vi "Request Frame.vi"(7 "Ignore Response":bool, 8 "error in (no error)":errorcluster, 9 "DA":u8, 10 "PGN":u32, 11 "Connection Info":T1) -> (0 "error out":errorcluster, 2 "Response Frame":T3 {"payload" format="%x"; "timestamp" format="%<%.7X\n%x>T"; "type" items=["CAN Data"=0, "CAN Remote"=1, "CAN Bus Error"=2, "CAN 2.0 Data"=8, "CAN FD Data"=16, "CAN FD+BRS Data"=24, "J1939 Data"=192, "Delay"=224, "Log Trigger"=225, "Start Trigger"=226]; "identifier" format="%x"}, 3 "Connection Info Out":T1)   [LabVIEW 2015, in "J1939 Addon Shared.lvlib"]
uses:
  J1939 Addon Shared.lvlib
  <vilib>/xnet/xnet.llb/XNET Frame CAN.ctl
  <vilib>/xnet/xnet.llb/XNET Frame Type CAN.ctl
  STM/TCP/stm_TCP Connection Info.ctl
  STM/_SubVIs/stm_MetaDataElement.ctl
  Types/Request Message.ctl
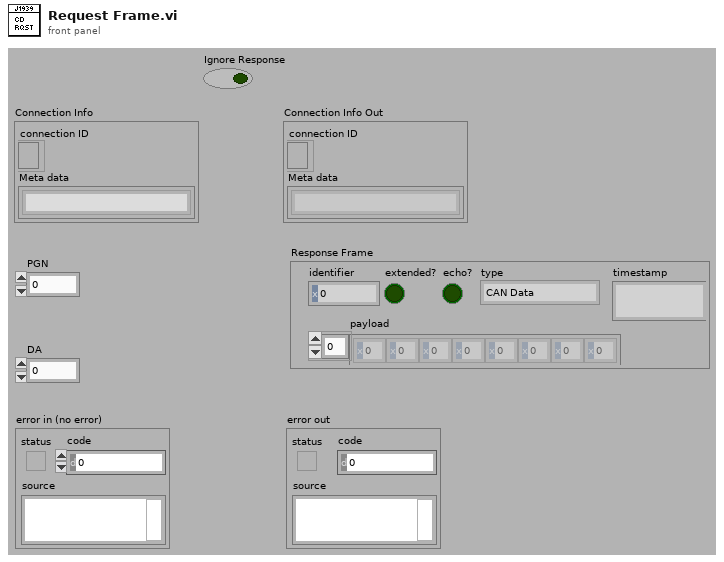
[diagram p1: front panel]
types:
  T1 = typedef "J1939 Addon Shared.lvlib/stm_TCP Connection Info.ctl" = cluster{"connection ID":refnum<k5>, "Meta data":T2[]}
  T2 = typedef "J1939 Addon Shared.lvlib/stm_MetaDataElement.ctl" = string
  T3 = typedef "XNET Frame CAN.ctl" = cluster{"timestamp":timestamp, "payload":u8[], "identifier":u32, "type":T4, "extended?":bool, "echo?":bool}
  T4 = typedef "XNET Frame Type CAN.ctl" = u8
  T5 = typedef "J1939 Addon Shared.lvlib/Request Message.ctl" = cluster{"PGN":u32, "DA":u8, "Ignore Response":bool}
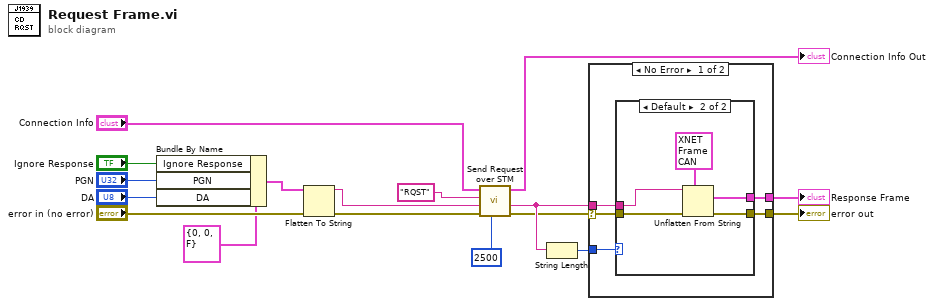
[diagram p0: block diagram]
diagram:
  n1 = Bundle By Name(cluster=T5 {"PGN"=0, "DA"=0, "Ignore Response"=FALSE} ("Cluster"), "Ignore Response"="Ignore Response", "PGN"="PGN", "DA"="DA") -> (w10:T5)
  n2 = Flatten To String(anything=w10, error in (no error)="error in (no error)") -> (data string=w6:string, error out=w5:errorcluster)  [unwired: 2 in, 1 out]
  n3 = call "Send Request over STM.vi"("Timeout (ms)"=2500 ("Timeout ms (5000)"), "error in (no error)"=w5, "Data"=w6, "Name"="RQST" ("Command"), "Connection Info"="Connection Info") -> ("error out"=w1:errorcluster, "Data"=w3:string, "Connection Info Out"=→"Connection Info Out":T1)  [unwired: 3 in, 1 out]
  n4 = String Length(string=w3) -> (length=w17:i32)
  n5 = case shown="No Error" w1 {
    selector: w1 -> [w19 w29]
    tunnel: [w22 w29] -> w14
    tunnel: w17 -> [w21 _]
    tunnel: w3 -> [w20 _]
    tunnel: [w18 _] -> w16
    frame No Error {
      n6 = case shown="Default" w21 {
        tunnel: w19 -> [w23 w27]
        tunnel: w20 -> [_ w24]
        tunnel: [w23 w26] -> w22
        tunnel: [_ w25] -> w18
        frame 0 {
        }
        frame Default {
          n7 = Unflatten From String(type=T3 {"timestamp"=timestamp(0 s since 1904-01-01), "payload"=[], "identifier"=0, "type"=0, "extended?"=FALSE, "echo?"=FALSE} ("element"), binary string=w24, error in (no error)=w27) -> (value=w25:T3, error out=w26:errorcluster)  [unwired: 2 in, 1 out]
        }
      }
    }
    frame Error {
    }
  }
  "Response Frame" <- w16
  "error out" <- w14
